vi "To String.vi"(8 "error in (no error)":errorcluster, 11 "Booleans in":refnum<class "Abs_Boolean.lvclass">) -> (0 "error out":errorcluster, 2 "String":string, 3 "Booleans out":refnum<class "Abs_Boolean.lvclass">)   [LabVIEW 2021, in "Abs_Boolean.lvclass"]
uses:
  Abs_Boolean.lvclass
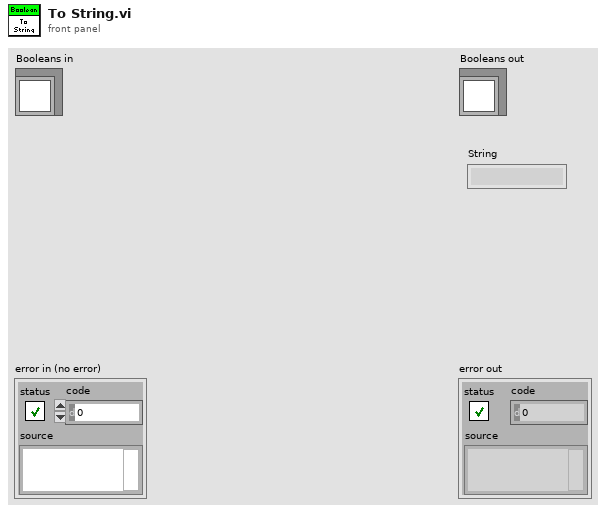
[diagram p1: front panel]
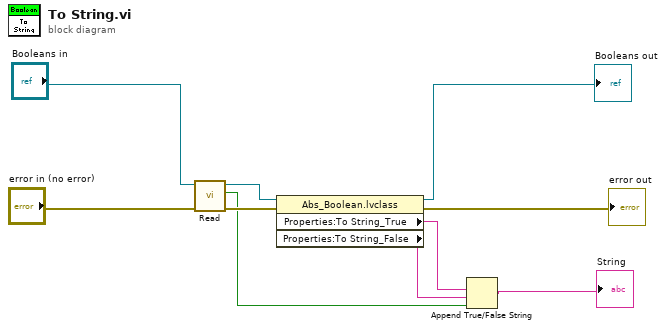
[diagram p0: block diagram]
diagram:
  n1 = call-dynamic "Read.vi"("error in (no error)"="error in (no error)", "Boolean in"="Booleans in") -> ("error out"=w4:errorcluster, "Boolean"=w3:bool, "Boolean out"=w5:refnum<class "Abs_Boolean.lvclass">)  [unwired: 7 in]
  n2 = property class="Abs_Boolean.lvclass"(reference=w5, error in=w4) -> (reference out=→"Booleans out":refnum<class "Abs_Boolean.lvclass">, error out=→"error out":errorcluster, "Properties:To String_True"=w2:string, "Properties:To String_False"=w1:string)
  n3 = Append True/False String(1:w3, 2:w1, 3:w2) -> (0:→"String":string)  [unwired: 1 in]
